vi "Save Engine.vi"(2 "Convert to U16?":bool, 5 "file path":path, 7 "#A-lines to save":u32, 9 "#Z pixels to save":u32, 11 "error in (no error)":errorcluster, 12 "Records Per Buffer":u32, 13 "pixels per record":u32) -> (4 "# elements in save queue":i32, 15 "error out":errorcluster)   [LabVIEW 2018]
uses:
  Controls/data manager action.ctl
  Controls/Queue Manager Actions.ctl
  Controls/QueueNames.ctl
  Controls/MessagePacket.ctl
  Controls/FGV Actions.ctl
  type defines/file type.ctl
panel:
  in  "File Type":T1
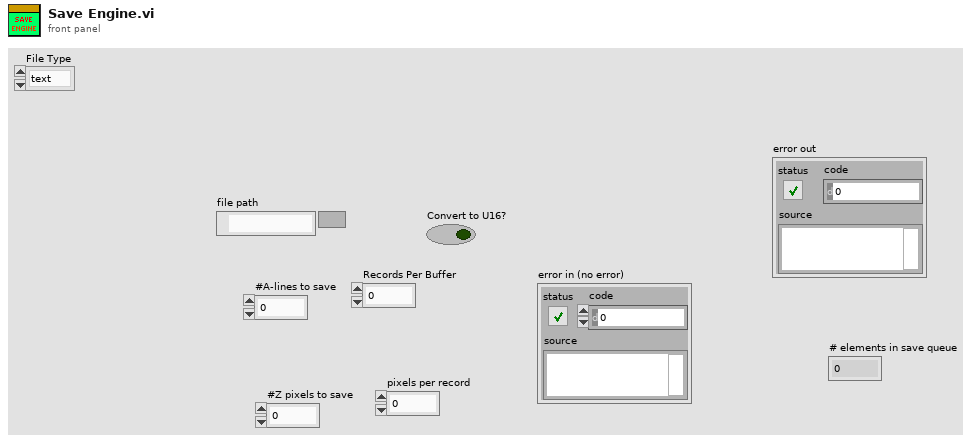
[diagram p1: front panel]
types:
  T1 = typedef "file type.ctl" = enum16{"text", "Tiff", "binary"}
  T2 = typedef "FGV Actions.ctl" = enum16{"Init", "Set", "Get", "Clear"}
  T3 = typedef "MessagePacket.ctl" = cluster{"Message":string, "Parameter":variant}
  T4 = typedef "QueueNames.ctl" = enum16{"Main GUI", "Main Scan Processor", "Main Processing", "Main Saving", "Main Display", "Main Table Stage GUI", "Main Table Stage Proc.", "Scan Engine", "Vibratome GUI", "Vibratome Processor", "Slice Engine"}
  T5 = typedef "Queue Manager Actions.ctl" = enum16{"Init", "Enqueue", "Enqueue All", "Preview Queue", "Dequeue", "Get Status", "Flush Queue", "Flush All Queues", "Release All Queues", "Release Queue", "Enqueue at Opposite End"}
  T6 = typedef "data manager action.ctl" = enum16{"Init: open file", "save", "save as text", "Uninit: close file"}
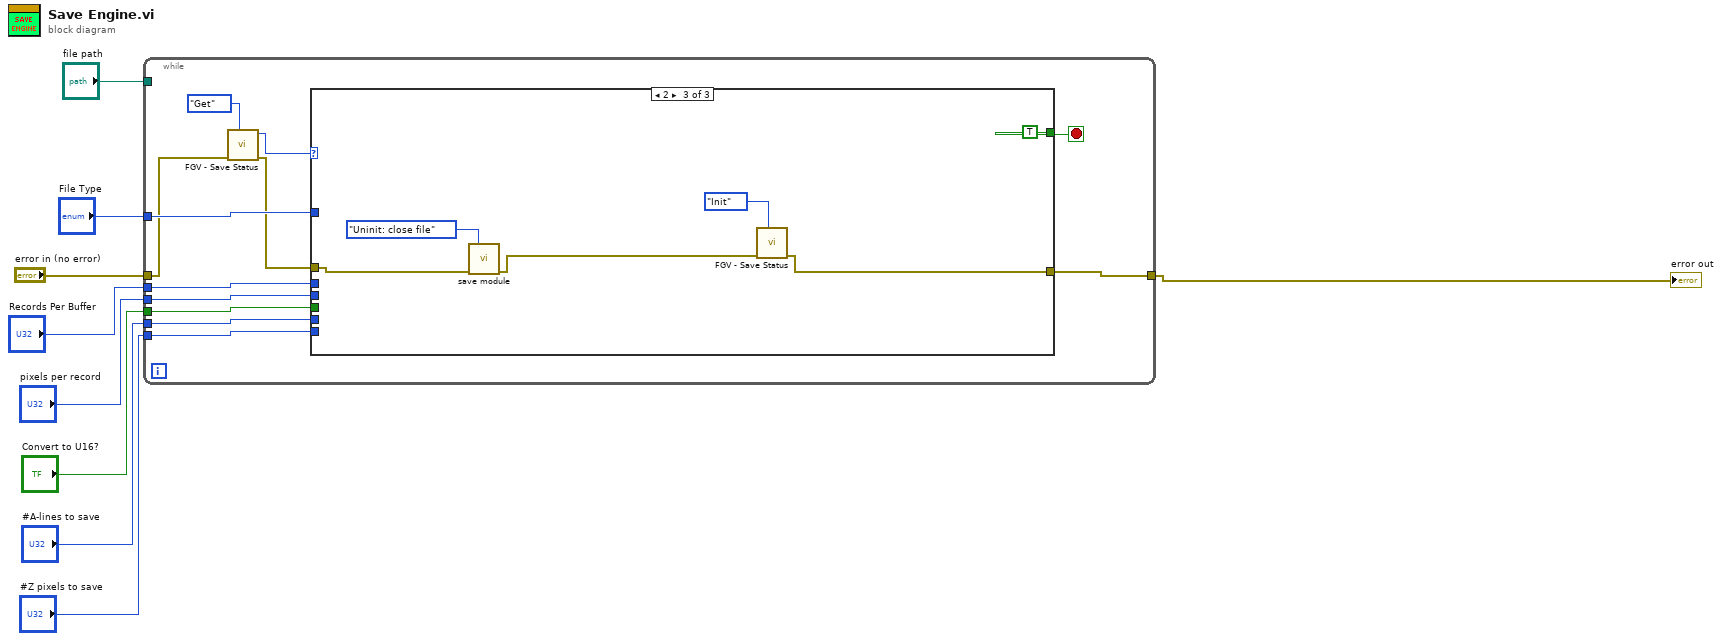
[diagram p0: block diagram]
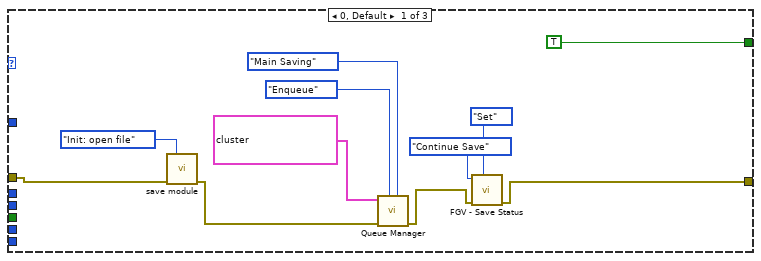
[diagram p2: hidden frame]
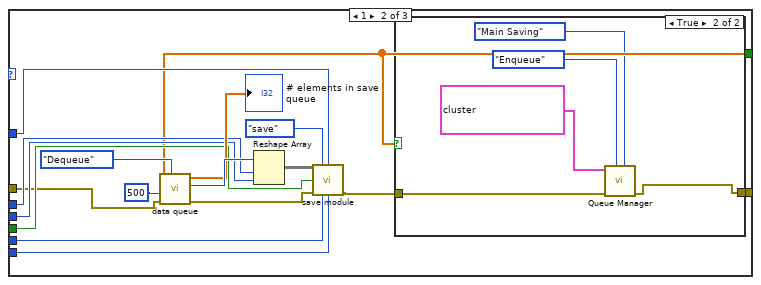
[diagram p3: hidden frame]
diagram:
  n1 = while {
    tunnel: "error in (no error)" -> [w11]
    tunnel: [w21] -> w1
    tunnel: "File Type" -> [w14]
    tunnel: "file path" -> [_]
    tunnel: "#A-lines to save" -> [w18]
    tunnel: "#Z pixels to save" -> [w19]
    tunnel: "Records Per Buffer" -> [w17]
    tunnel: "pixels per record" -> [w16]
    tunnel: "Convert to U16?" -> [w15]
    stop <- w20 stop-if-true
    n2 = call "FGV - Save Status.vi"("Actions"=FGV_Actions."Get", "Error In"=w11) -> ("Error Out"=w10:errorcluster, "Save Status out"=w12:u16)  [unwired: 7 in, 1 out]
    n3 = case shown="2" w12 {
      tunnel: [w26 w34 w59] -> w21
      tunnel: [TRUE ("Empty?") w36 TRUE ("Empty?")] -> w20
      tunnel: w19 -> [_ w42 _]
      tunnel: w18 -> [_ w41 _]
      tunnel: w17 -> [_ w40 _]
      tunnel: w16 -> [_ w39 _]
      tunnel: w15 -> [_ w38 _]
      tunnel: w14 -> [_ w37 _]
      tunnel: w10 -> [w22 w33 w56]
      frame 0, Default {
        n4 = call "save module.vi"("action"=data_manager_action."Init: open file", "error in (no error)"=w22) -> ("error out"=w28:errorcluster)  [unwired: 12 in, 1 out]
        n5 = call "Queue Manager.vi"("Queue Name"=QueueNames."Main Saving", "Action"=Queue_Manager_Actions."Enqueue", "Error In"=w28, "Message Packet Array"=T3[] [{"Message"="Save", "Parameter"=variant}, {"Message"="Saving", "Parameter"=variant}, {"Message"="", "Parameter"=variant}]) -> ("Error Out"=w27:errorcluster)  [unwired: 3 in, 4 out]
        n6 = call "FGV - Save Status.vi"("Actions"=FGV_Actions."Set", "Error In"=w27, "Save Status in"=enum16{"Start", "Continue Save", "Finish Save"}."Continue Save") -> ("Error Out"=w26:errorcluster)  [unwired: 6 in, 2 out]
      }
      frame 1 {
        n7 = call "data queue.vi"("Action"=Queue_Manager_Actions."Dequeue", "error in (no error)"=w33, 9:500 ("timeout in ms (-1)")) -> ("error out"=w43:errorcluster, "# elements in queue"=w47:i32, "data out"=→"# elements in save queue":sgl[], "data in"=w36:sgl[])  [unwired: 4 in, 1 out]
        n8 = Reshape Array(w47, w40, w39) -> (w44:void[][])
        n9 = call "save module.vi"("data in"=w44, "action"=data_manager_action."save", "File Type"=w37, "Convert to U16?"=w38, "error in (no error)"=w43, "# A-lines to save"=w41, "#Z pixels to save"=w42) -> ("error out"=w35:errorcluster)  [unwired: 7 in, 1 out]
        n10 = case shown="True" w36 {
          tunnel: w35 -> [w50 w52]
          tunnel: [w50 w51] -> w34
          frame False {
          }
          frame True {
            n11 = call "Queue Manager.vi"("Queue Name"=QueueNames."Main Saving", "Action"=Queue_Manager_Actions."Enqueue", "Error In"=w52, "Message Packet Array"=T3[] [{"Message"="Save", "Parameter"=variant}, {"Message"="Saving", "Parameter"=variant}, {"Message"="", "Parameter"=variant}]) -> ("Error Out"=w51:errorcluster)  [unwired: 3 in, 4 out]
          }
        }
      }
      frame 2 {
        n12 = call "save module.vi"("action"=data_manager_action."Uninit: close file", "error in (no error)"=w56) -> ("error out"=w60:errorcluster)  [unwired: 12 in, 1 out]
        n13 = call "FGV - Save Status.vi"("Actions"=FGV_Actions."Init", "Error In"=w60) -> ("Error Out"=w59:errorcluster)  [unwired: 7 in, 2 out]
      }
    }
  }
  "error out" <- w1
